vi "FGV_Included_File Extensions.vi"() -> (3 "Included File Extensions (Lower Case)":string[](array[string]))   [LabVIEW 2019]
uses:
  AutoMenuCreator.lvlib
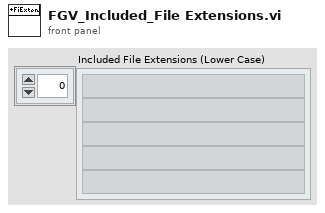
[diagram p1: front panel]
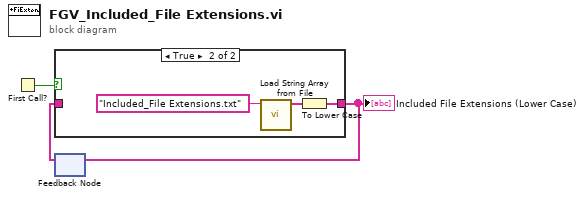
[diagram p0: block diagram]
diagram:
  n1 = First Call?() -> (First Call?: T/F=w3:bool)
  n2 = feedback #1() -> (w1:string[])  [unwired: 1 in]
  n3 = case shown="True" w3 {
    tunnel: [w4 w5] -> w2
    tunnel: w1 -> [w4 _]
    frame False {
    }
    frame True {
      n4 = call "Load String Array from File.vi"("File name"="Included_File Extensions.txt") -> ("Loaded 1D String Array"=w6:string[])  [unwired: 9 in, 1 out]
      n5 = To Lower Case(string=w6) -> (all lower case string=w5:string[])
    }
  }
  "Included File Extensions (Lower Case)" <- w2
  n6 = feedback-in #1(w2) -> ()
